vi "ConfigTrigger.vi"(8 "error in (no error)":errorcluster, 11 "DigitizerBase in":refnum<class "DigitizerBase.lvclass">) -> (0 "error out":errorcluster, 3 "DigitizerBase out":refnum<class "DigitizerBase.lvclass">)   [LabVIEW 2014, in "DigitizerPlugins.lvlib" / "DigitizerBase.lvclass"]
uses:
  DigitizerBase.lvclass
  DigitizerBase.lvclass/DigitizerBase.ctl
  Accessors/Read InstRef.vi
  Accessors/Read Trigger.vi
  Accessors/Read Sources.vi
  Accessors/Write InstRef.vi
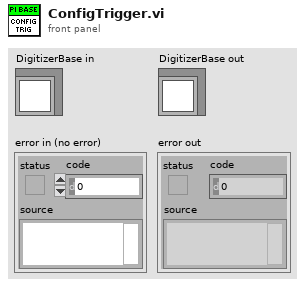
[diagram p1: front panel]
types:
  T1 = typedef "DigitizerPlugins.lvlib/DigitizerBase.lvclass/Trigger.ctl" = cluster{"Source":string, "Delay":dbl, "Holdoff":dbl, "PretriggerSamples":i32, "Sources":T2[]}
  T2 = typedef "DigitizerPlugins.lvlib/DigitizerBase.lvclass/TrigSource.ctl" = cluster{"Name":string, "Coupling":enum16{"AC", "DC", "HF Reject", "LF Reject", "Noise Reject"}, "Hysteresis":dbl, "Level":dbl, "Slope":enum16{"Positive", "Negative"}, "Type":enum16{"Edge", "Width", "Runt", "Glitch", "TV", "Window"}}
  T3 = enum16{"Edge", "Width", "Runt", "Glitch", "TV", "Window"}
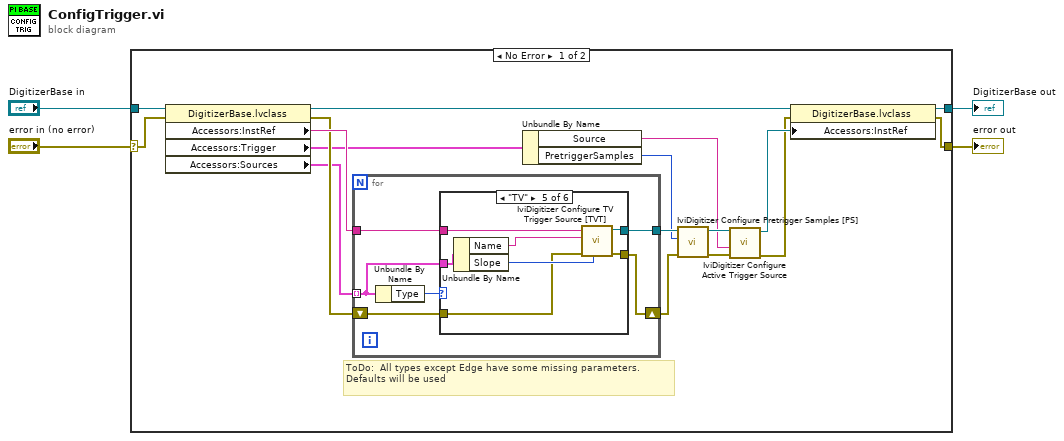
[diagram p0: block diagram]
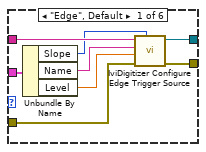
[diagram p2: hidden frame]
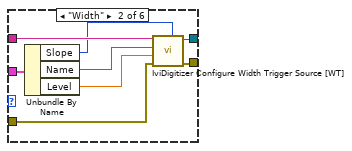
[diagram p3: hidden frame]
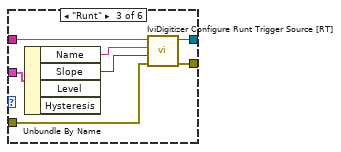
[diagram p4: hidden frame]
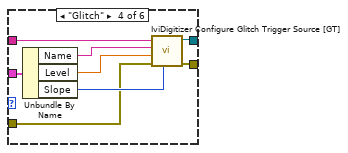
[diagram p5: hidden frame]
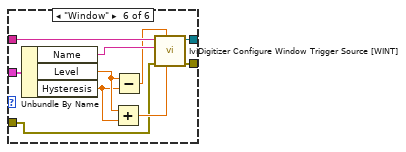
[diagram p6: hidden frame]
diagram:
  n1 = case shown="No Error" "error in (no error)" {
    selector: "error in (no error)" -> [w19 w77]
    tunnel: [w5 w77] -> w3
    tunnel: [w8 w76] -> w1
    tunnel: "DigitizerBase in" -> [w21 w76]
    frame No Error {
      # "ToDo:  All types except Edge have some missing parameters. Defaults will be used"
      n2 = property class="DigitizerBase.lvclass"(reference=w21, error in=w19) -> (reference out=w20:refnum<class "DigitizerBase.lvclass">, error out=w17:errorcluster, "Accessors:InstRef"=w18:string, "Accessors:Trigger"=w15:T1, "Accessors:Sources"=w16:T2[])
      n3 = for {
        tunnel: w16 -> [w26] mode=indexing
        tunnel: w18 -> [w25]
        shift-right: [w23] -> w13
        shift-left: w17 -> [w24]
        tunnel: [w22] -> w14
        n4 = Unbundle By Name(w26) -> ("Type"=w27:T3)
        n5 = case shown="\"TV\"" w27 {
          tunnel: w26 -> [w34 w42 w48 w56 w63 w73]
          tunnel: w25 -> [w35 w43 w49 w57 w64 w74]
          tunnel: w24 -> [w30 w38 w45 w52 w60 w67]
          tunnel: [w29 w37 w50 w58 w65 w75] -> w23
          tunnel: [w28 w36 w44 w51 w59 w66] -> w22
          frame "Edge", Default {
            n6 = Unbundle By Name(w34) -> ("Slope"=w33:enum16{"Positive", "Negative"}, "Name"=w32:string, "Level"=w31:dbl)
            n7 = call <vilib>:"IviDigitizer Configure Edge Trigger Source.vi"("Trigger Slope (Positive)"=w33, "error in (no error)"=w30, "Trigger Level (1.0)"=w31, "Trigger Source (\"\")"=w32, "instrument handle"=w35) -> ("error out"=w29:errorcluster, "instrument handle out"=w28:refnum<k15>)  [unwired: 5 in]
          }
          frame "Width" {
            n8 = Unbundle By Name(w42) -> ("Slope"=w40:enum16{"Positive", "Negative"}, "Name"=w41:string, "Level"=w39:dbl)
            n9 = call <vilib>:"IviDigitizer Configure Width Trigger Source [WT].vi"("Width Polarity (Positive)"=w40, "error in (no error)"=w38, "Trigger Level (1.0)"=w39, "Trigger Source (\"\")"=w41, "instrument handle"=w43) -> ("error out"=w37:errorcluster, "instrument handle out"=w36:refnum<k15>)  [unwired: 5 in]
          }
          frame "Runt" {
            n10 = Unbundle By Name(w48) -> ("Name"=w47:string, "Slope"=w46:enum16{"Positive", "Negative"})  [unwired: 2 out]
            n11 = call <vilib>:"IviDigitizer Configure Runt Trigger Source [RT].vi"("error in (no error)"=w45, "Runt Polarity (Positive)"=w46, "Trigger Source (\"\")"=w47, "instrument handle"=w49) -> ("error out"=w50:errorcluster, "instrument handle out"=w44:refnum<k15>)  [unwired: 6 in]
          }
          frame "Glitch" {
            n12 = Unbundle By Name(w56) -> ("Name"=w55:string, "Level"=w54:dbl, "Slope"=w53:enum16{"Positive", "Negative"})
            n13 = call <vilib>:"IviDigitizer Configure Glitch Trigger Source [GT].vi"("Glitch Polarity (Positive)"=w53, "error in (no error)"=w52, "Trigger Level (1.0)"=w54, "Trigger Source (\"\")"=w55, "instrument handle"=w57) -> ("error out"=w58:errorcluster, "instrument handle out"=w51:refnum<k15>)  [unwired: 5 in]
          }
          frame "TV" {
            n14 = Unbundle By Name(w63) -> ("Name"=w62:string, "Slope"=w61:enum16{"Positive", "Negative"})
            n15 = call <vilib>:"IviDigitizer Configure TV Trigger Source [TVT].vi"("TV Polarity (Positive)"=w61, "error in (no error)"=w60, "Trigger Source (\"\")"=w62, "instrument handle"=w64) -> ("error out"=w65:errorcluster, "instrument handle out"=w59:refnum<k15>)  [unwired: 6 in]
          }
          frame "Window" {
            n16 = Unbundle By Name(w73) -> ("Name"=w72:string, "Level"=w70:dbl, "Hysteresis"=w69:dbl)
            n17 = Add(x=w70, y=w69) -> (x+y=w68:dbl)
            n18 = Subtract(x=w70, y=w69) -> (x-y=w71:dbl)
            n19 = call <vilib>:"IviDigitizer Configure Window Trigger Source [WINT].vi"("Threshold High (1.0)"=w68, "Threshold Low (1.0)"=w71, "error in (no error)"=w67, "Trigger Source (\"\")"=w72, "instrument handle"=w74) -> ("error out"=w75:errorcluster, "instrument handle out"=w66:refnum<k15>)  [unwired: 5 in]
          }
        }
      }
      n20 = Unbundle By Name(w15) -> ("Source"=w9:string, "PretriggerSamples"=w12:i32)
      n21 = call <vilib>:"IviDigitizer Configure Pretrigger Samples [PS].vi"("instrument handle"=w14, "Pretrigger Samples (1)"=w12, "error in (no error)"=w13) -> ("instrument handle out"=w10:refnum<k15>, "error out"=w11:errorcluster)  [unwired: 6 in]
      n22 = call <vilib>:"IviDigitizer Configure Active Trigger Source.vi"("error in (no error)"=w11, "Trigger Source (\"\")"=w9, "instrument handle"=w10) -> ("error out"=w6:errorcluster, "instrument handle out"=w7:refnum<k15>)  [unwired: 7 in]
      n23 = property class="DigitizerBase.lvclass"(reference=w20, error in=w6, "Accessors:InstRef"=w7) -> (reference out=w8:refnum<class "DigitizerBase.lvclass">, error out=w5:errorcluster)
    }
    frame Error {
    }
  }
  "error out" <- w3
  "DigitizerBase out" <- w1
